vi "sCMOS_main.vi"   [LabVIEW 2015]
uses:
  CONTROLS/Q_camera_element.ctl
  CONTROLS/Q_main_element.ctl
  <vilib>/vision/Image Controls.llb/IMAQ Image.ctl
  CONTROLS/Global parameters.ctl
  GLOBAL/Global_CAMERA.vi
  GLOBAL/Global_ABORT.vi
  GLOBAL/Global_MAIN.vi
types:
  T1 = typedef "Q_main_element.ctl" = cluster{"variant":variant, "Instruction":enum16{"Main_idle", "Main_initialize", "Main_initialize_TDMS", "Main_initialize_Queue", "Main_error", "Main_DAQ_initialization_results", "Main_ASI_initialization_results", "Main_Piezo_initialization_results", "Main_Valve_initialization_results", "Main_Pump_initialization_results", "Main_CAMERA_initialization_results", "Main_DAQ_error", "Main_ASI_error", "Main_Piezo_error", "Main_CAMERA_error", "Main_Valve_error", "Main_Pump_error", "Main_start_acquiring", "Main_not_acquiring", "Main_acquiring", "Main_stop_acquiring", "Main_change_exposure", "Main_change_z_scan_parameters", "Main_define_ROI", "Main_read_kinetic_time", "Main_cooler", "Main_read_temperature", "Main_save_XY", "Main_define_mosaic", "Main_load_XY", "Main_discard_XY", "Main_move_to_XY", "Main_measure_QPD", "Main_autofocus_calibration", "Main_save_PID", "Main_change_H_valve_position", "Main_two_way_valve", "Main_save_movie", "Main_init_single_scan", "Main_single_scan", "Main_stop_single_scan", "Main_merFISH_illumination_parameters", "Main_merFISH_buffer_probe_list", "Main_merFISH_injections_procedure", "Main_merFISH_save_setpoint", "Main_merFISH_DAPI_parameters", "Main_merFISH_Brightfield_parameters", "Main_merFISH_save_embryo_ROI", "Main_merFISH_init", "Main_merFISH_resume", "Main_merFISH_start_autofocus", "Main_merFISH_open_close_valve_merFISH", "Main_merFISH_open_close_valve_photobleaching", "Main_merFISH_hybridization", "Main_merFISH_move_to_ROI", "Main_merFISH_wait_stabilization", "Main_merFISH_scan_laser", "Main_merFISH_scan_brightfield", "Main_merFISH_photobleaching_injection", "Main_merFISH_photobleaching", "Main_merFISH_save", "Main_merFISH_send_email", "Main_merFISH_close", "Main_TL_define_parameters", "Main_TL_FTL_reset_parameters", "Main_TL_init", "Main_TL_start_autofocus", "Main_TL_move_to_ROI", "Main_TL_wait_for_stabilization", "Main_TL_scan", "Main_TL_wait_cycle_end", "Main_TL_close", "Main_FTL_define_parameters", "Main_FTL_init", "Main_STOP"}}
  T2 = typedef "Image Type" = u32
  T3 = typedef "Q_camera_element.ctl" = cluster{"variant":variant, "Instruction":enum16{"CAMERA_idle", "CAMERA_initialize", "CAMERA_error", "CAMERA_security_stop", "CAMERA_not_acquiring", "CAMERA_acquiring", "CAMERA_start_acquiring", "CAMERA_stop_acquiring", "CAMERA_change_exposure", "CAMERA_define_ROI", "CAMERA_cooler", "CAMERA_acquire_movie", "CAMERA_init_scan", "CAMERA_check_new_scan_image", "CAMERA_close_scan", "CAMERA_init_merFISH", "CAMERA_start_acquiring_merFISH", "CAMERA_close_scan_merFISH", "CAMERA_close_merFISH", "CAMERA_init_TL", "CAMERA_start_acquiring_TL", "CAMERA_stop_acquiring_TL", "CAMERA_close_TL", "CAMERA_STOP"}}
  T4 = typedef "IMAQ Image.ctl" = refnum<image>
  T5 = cluster{"Total kinetic time (s)":dbl, "temperature":dbl, "coolerStatus":i32, "Error":bool, "Real time image":T4}
  T6 = cluster{"Exposure time":dbl, "Start acquisition":bool}
  T7 = cluster{"Sub Region":cluster{"Horizontal Offset":i32, "Vertical Offset":i32, "Horizontal Size":i32, "Vertical Size":i32}, "Start acquisition":bool}
  T8 = typedef "Global parameters.ctl" = cluster{"405":dbl, "488":dbl, "561":dbl, "641":dbl, "BF":dbl, "X":dbl, "Y":dbl, "Filter list":u16, "Exp time":sgl, "Kinetic time":sgl, "Gain":i32, "Step length (nm)":u32, "Total range (nm)":u32, "Scan illumination\n mode":bool, "Dt (s)":i32, "# repetitions":i32}
  T9 = cluster{"Saving path":path, "Sample name":string, "N frames":i32, "N movies":i32, "Start acquisition":bool, "Global parameters":T8}
  T10 = cluster{"Frames":i32, "Movie path":path, "Start acquisition":bool}
  T11 = cluster{"Pulse length Ton (s)":dbl, "image #":i32, "Display?":bool}
  T12 = cluster{"Mode":u32, "Polarity":u32, "Times":u32, "Delay":dbl}
  T13 = enum16{"CAMERA_idle", "CAMERA_initialize", "CAMERA_error", "CAMERA_security_stop", "CAMERA_not_acquiring", "CAMERA_acquiring", "CAMERA_start_acquiring", "CAMERA_stop_acquiring", "CAMERA_change_exposure", "CAMERA_define_ROI", "CAMERA_cooler", "CAMERA_acquire_movie", "CAMERA_init_scan", "CAMERA_check_new_scan_image", "CAMERA_close_scan", "CAMERA_init_merFISH", "CAMERA_start_acquiring_merFISH", "CAMERA_close_scan_merFISH", "CAMERA_close_merFISH", "CAMERA_init_TL", "CAMERA_start_acquiring_TL", "CAMERA_stop_acquiring_TL", "CAMERA_close_TL", "CAMERA_STOP"}
  T14 = cluster{"Horizontal Offset":i32, "Vertical Offset":i32, "Horizontal Size":i32, "Vertical Size":i32}
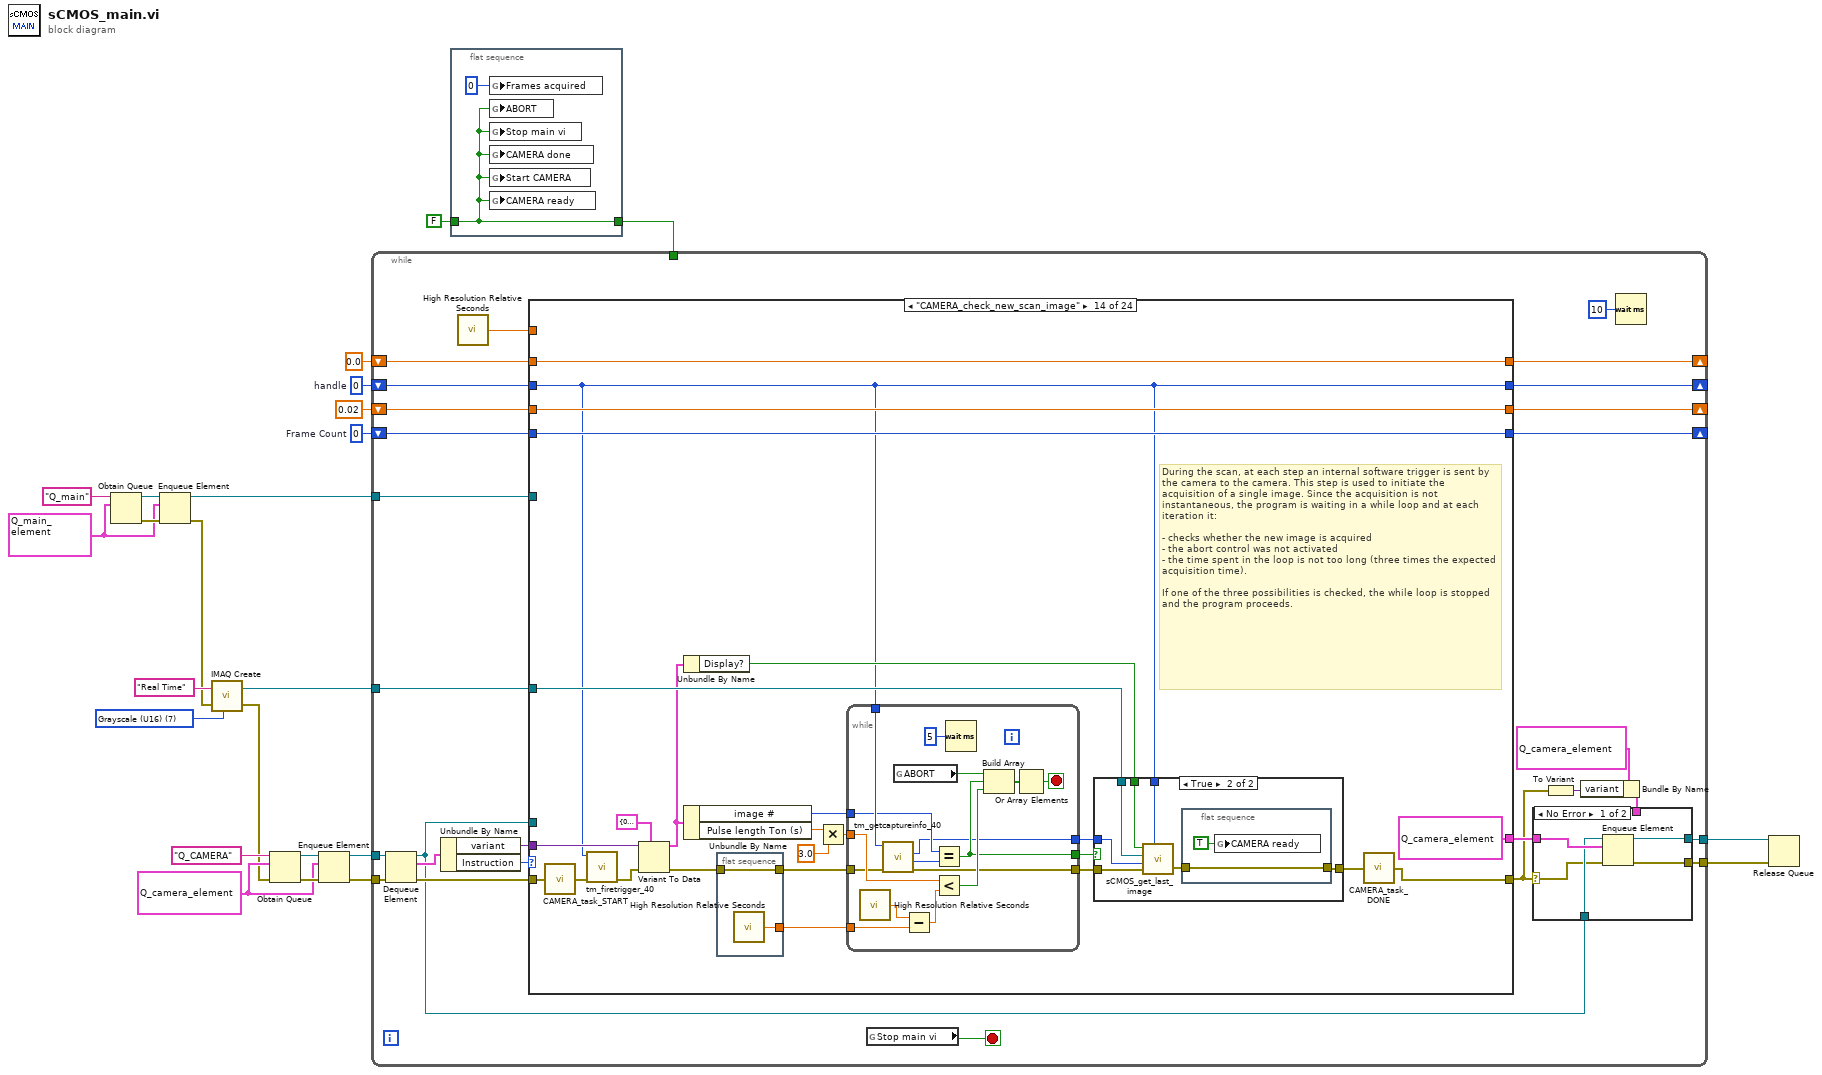
[diagram p0: block diagram]
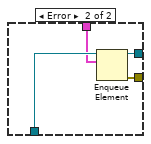
[diagram p2: hidden frame]
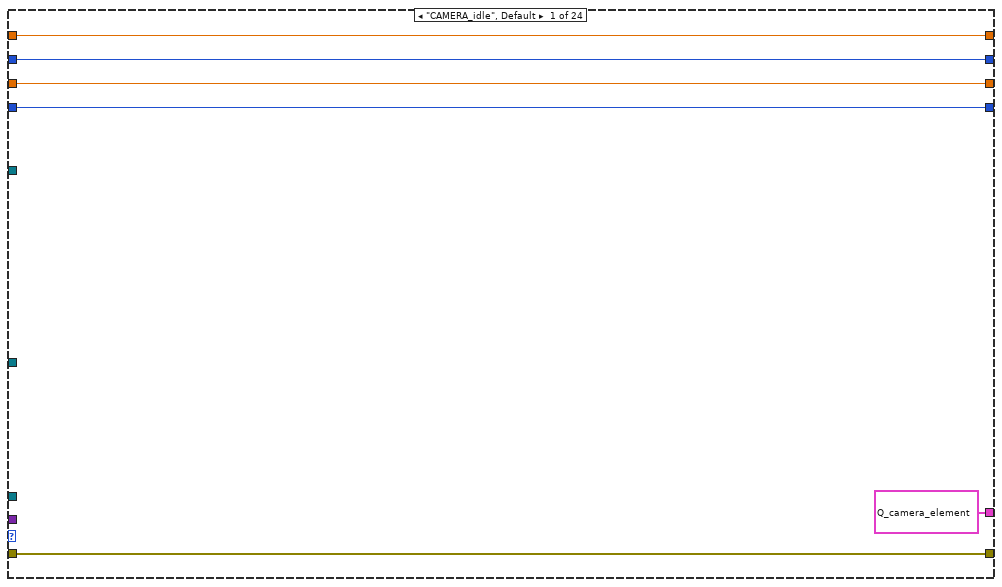
[diagram p3: hidden frame]
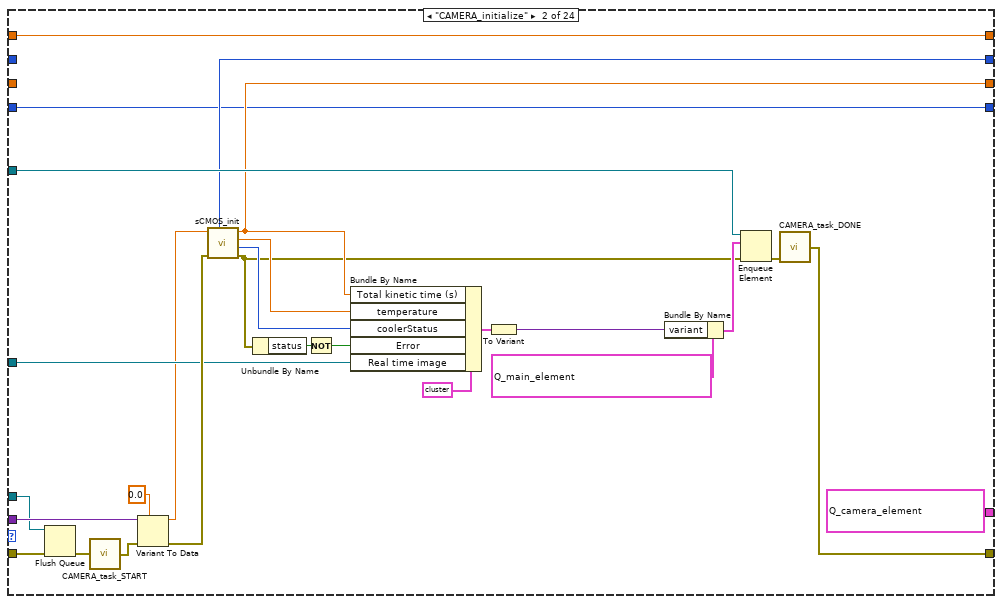
[diagram p4: hidden frame]
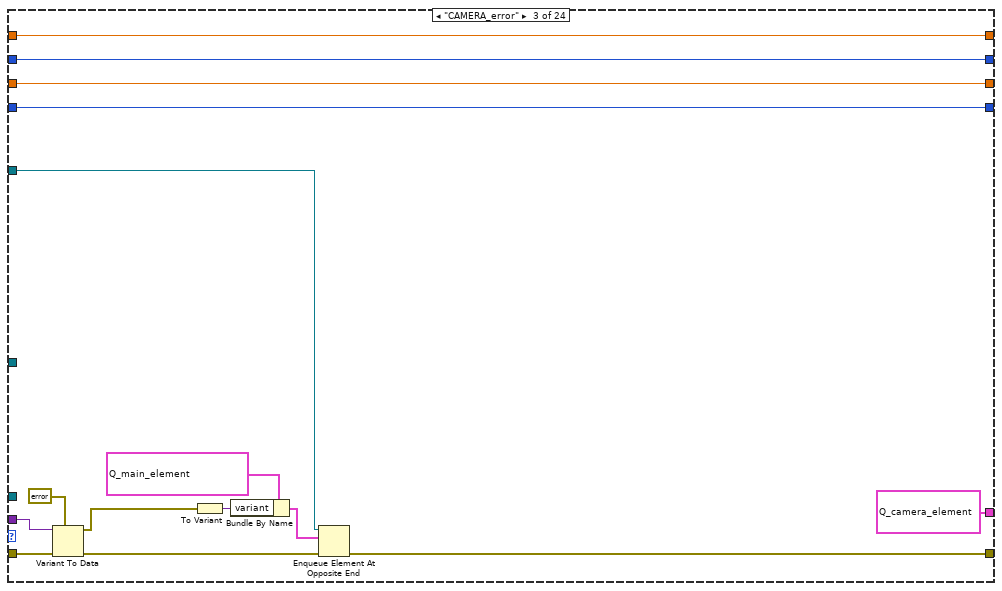
[diagram p5: hidden frame]
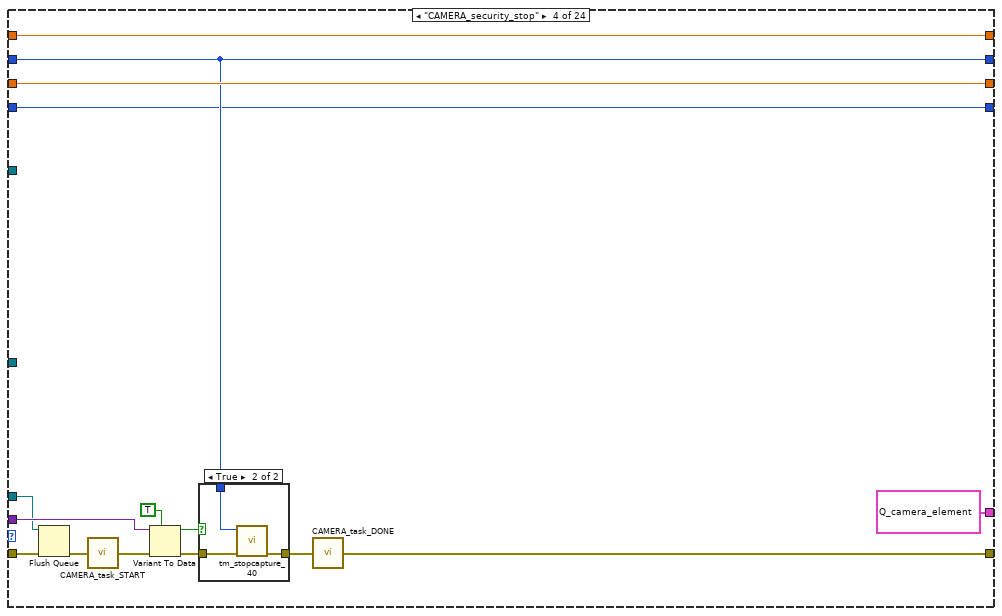
[diagram p6: hidden frame]
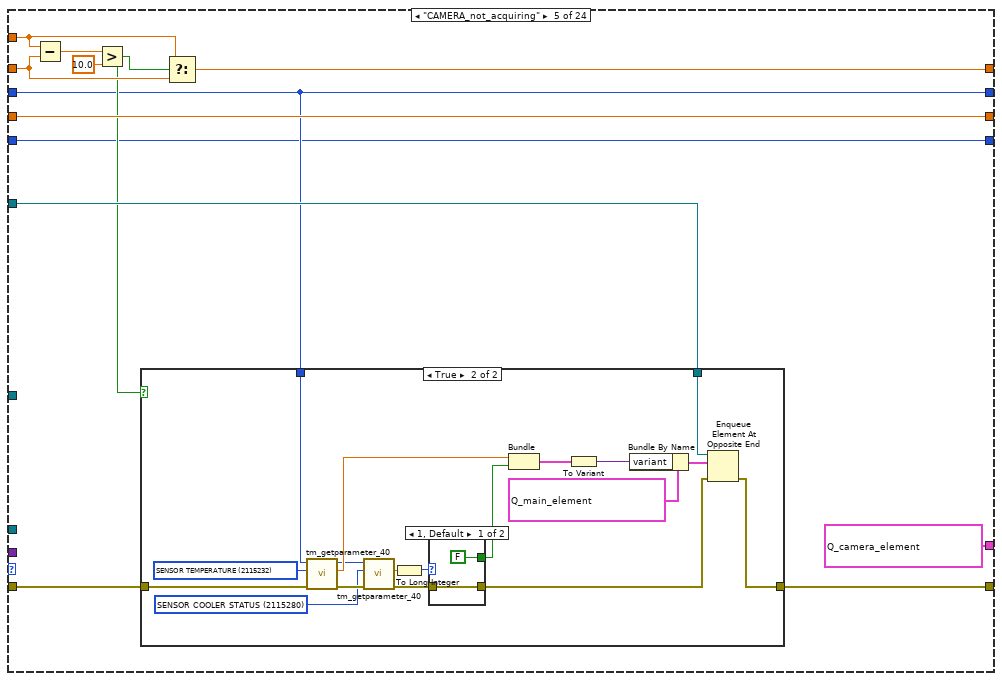
[diagram p8: hidden frame]
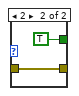
[diagram p10: hidden frame]
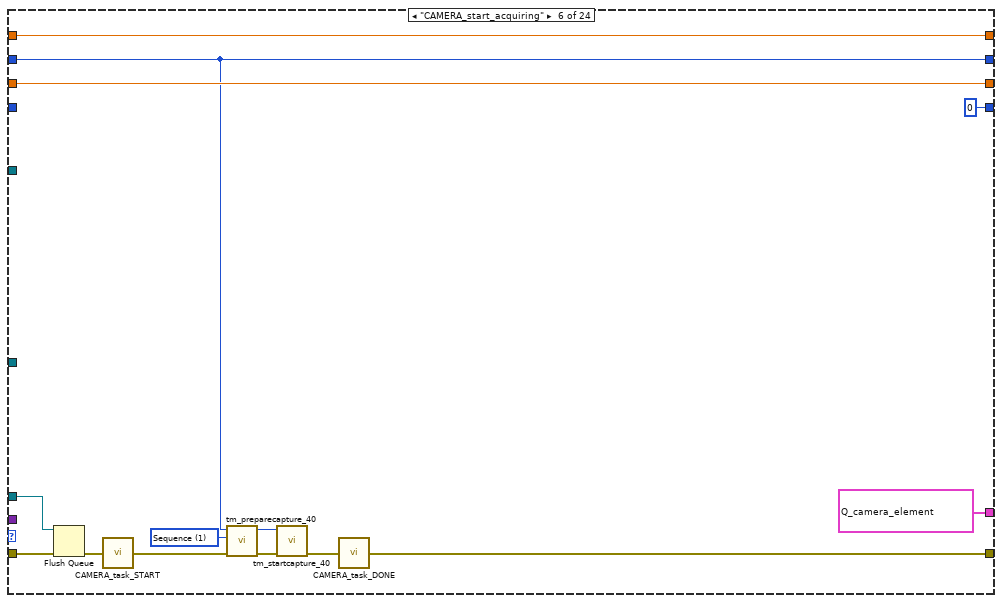
[diagram p11: hidden frame]
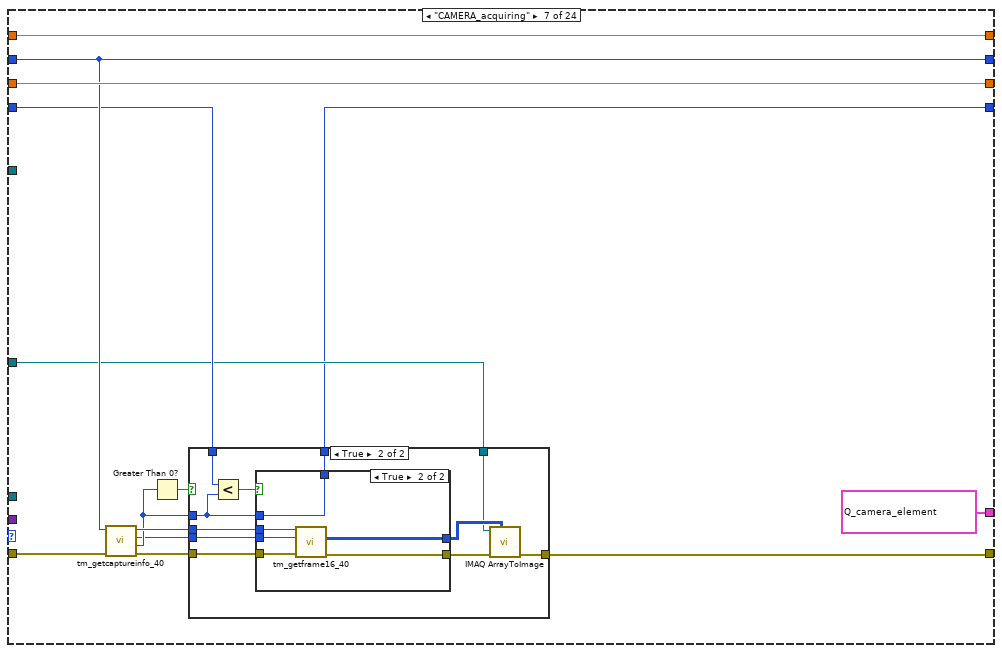
[diagram p12: hidden frame]
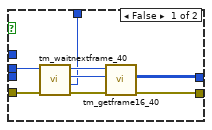
[diagram p14: hidden frame]
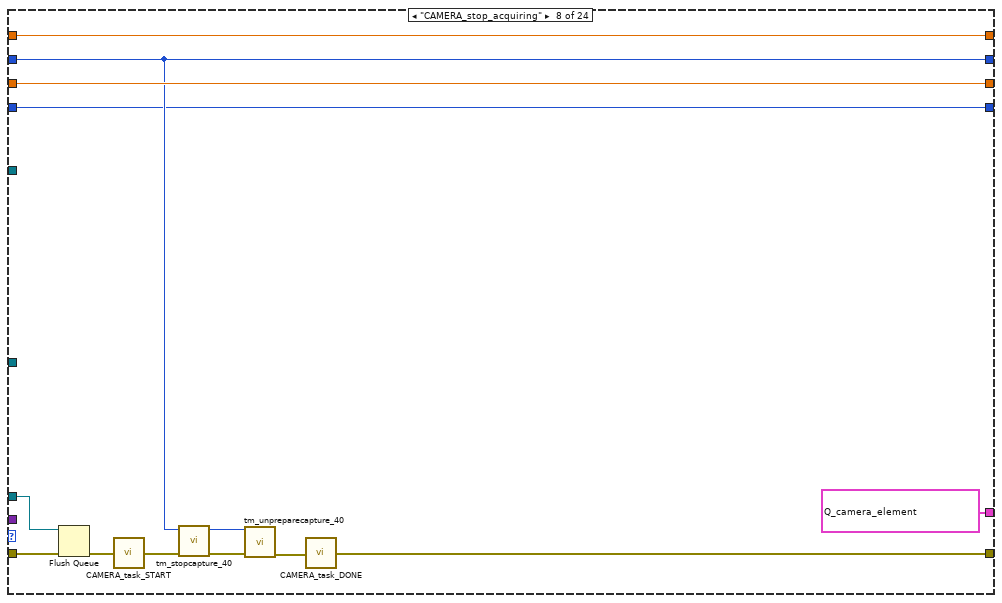
[diagram p15: hidden frame]
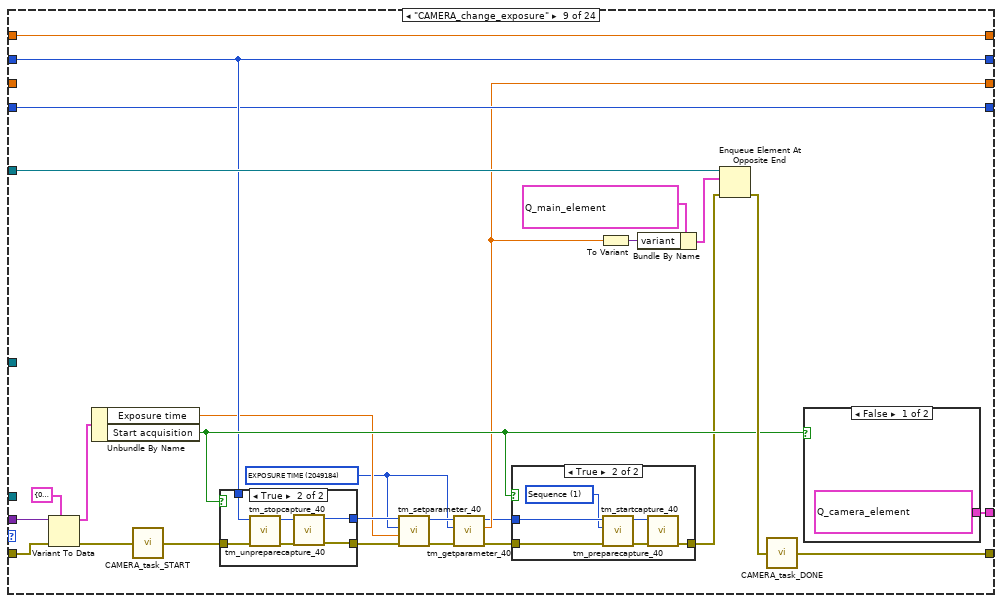
[diagram p16: hidden frame]
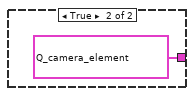
[diagram p18: hidden frame]
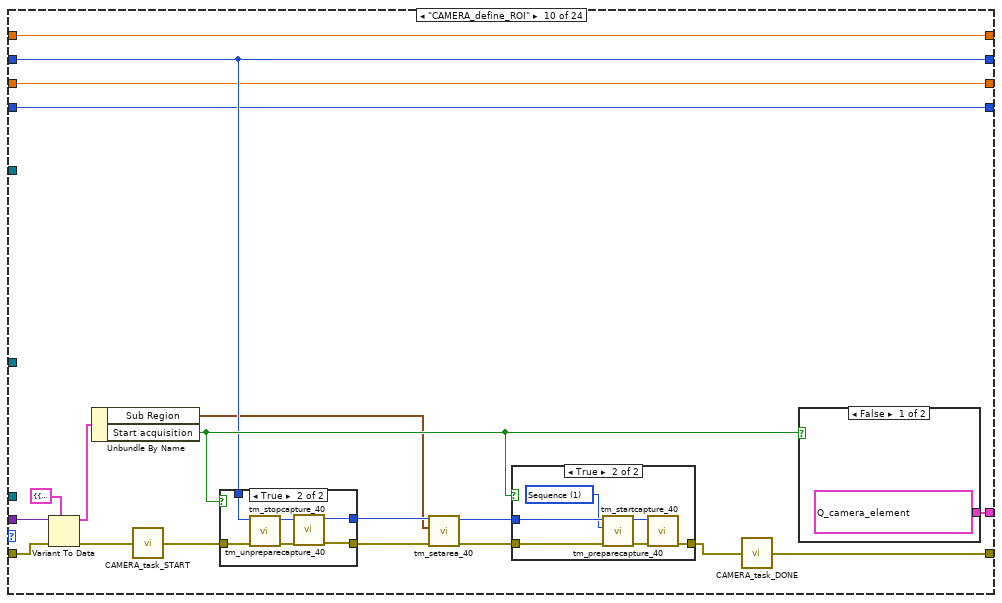
[diagram p20: hidden frame]
diagram:
  w1 = 0  # Frame Count
  w2 = u32 0  # handle
  w3 = T1 {"variant"=variant, "Instruction"=enum."Main_idle"} ("Q_main_element")
  w14 = T2 7 items=["Grayscale (U8)", "Grayscale (I16)", "Grayscale (SGL)", "Complex (CSG)", "RGB (U32)", "HSL (U32)", "RGB (U64)", "Grayscale (U16)"] ("Image Type")
  w19 = T3 {"variant"=variant, "Instruction"=enum."CAMERA_idle"} ("Q_ANDOR_element")
  n1 = Obtain Queue(name (unnamed)="Q_main", element data type=w3) -> (queue out=w17:refnum<queue>, error out=w18:errorcluster)  [unwired: 3 in, 1 out]
  n2 = Enqueue Element(queue=w17, element=w3, error in (no error)=w18) -> (queue out=w16:refnum<queue>, error out=w13:errorcluster)  [unwired: 1 in, 1 out]
  n3 = call "IMAQ Create"("Image Name"="Real Time", "Image Type"=w14, "error in (no error)"=w13) -> ("New Image"=w12:T4, "error out"=w9:errorcluster)  [unwired: 2 in]
  n4 = Obtain Queue(name (unnamed)="Q_CAMERA", element data type=w19, error in (no error)=w9) -> (queue out=w23:refnum<queue>, error out=w22:errorcluster)  [unwired: 2 in, 1 out]
  n5 = Enqueue Element(queue=w23, element=w19, error in (no error)=w22) -> (queue out=w21:refnum<queue>, error out=w20:errorcluster)  [unwired: 1 in, 1 out]
  n6 = while {
    tunnel: w21 -> [w50]
    tunnel: w20 -> [w49]
    tunnel: [w44] -> w6
    tunnel: w16 -> [w43]
    tunnel: w12 -> [w41]
    shift-right: [w39] -> _
    shift-left: 0.02 -> [w40]
    shift-right: [w38] -> _
    shift-left: 0.0 ("Period") -> [w37]
    tunnel: w7 -> [_]
    tunnel: [w36] -> w5
    shift-right: [w30] -> _
    shift-left: w2 -> [w31]
    shift-right: [w28] -> _
    shift-left: w1 -> [w29]
    stop <- w51 stop-if-true
    n7 = Dequeue Element(queue=w50, error in (no error)=w49) -> (queue out=w25:refnum<queue>, element=w48:T3, error out=w46:errorcluster)  [unwired: 1 in, 1 out]
    n8 = Unbundle By Name(w48) -> ("variant"=w42:variant, "Instruction"=w47:T13)
    n9 = call <vilib>:"High Resolution Relative Seconds.vi"() -> ("relative seconds"=w27:dbl)
    n10 = case shown="\"CAMERA_check_new_scan_image\"" w47 {
      tunnel: w46 -> [w64 w79 w107 w111 w138 w173 w188 w228 w257 w293 w328 w347 w398 w424 w474 w490 w510 w529 w548 w566 w591 w610 w632 w650]
      tunnel: [w64 w75 w94 w120 w137 w174 w180 w227 w250 w289 w323 w345 w397 w416 w475 w489 w513 w530 w549 w565 w590 w609 w633 w648] -> w33
      tunnel: [T3 {"variant"=variant, "Instruction"=enum."CAMERA_idle"} ("Q_ANDOR_element") T3 {"variant"=variant, "Instruction"=enum."CAMERA_not_acquiring"} ("Q_ANDOR_element") T3 {"variant"=variant, "Instruction"=enum."CAMERA_idle"} ("Q_ANDOR_element") T3 {"variant"=variant, "Instruction"=enum."CAMERA_idle"} ("Q_ANDOR_element") T3 {"variant"=variant, "Instruction"=enum."CAMERA_not_acquiring"} ("Q_ANDOR_element") T3 {"variant"=variant, "Instruction"=enum."CAMERA_acquiring"} ("Q_ANDOR_element") T3 {"variant"=variant, "Instruction"=enum."CAMERA_acquiring"} ("Q_ANDOR_element") T3 {"variant"=variant, "Instruction"=enum."CAMERA_not_acquiring"} ("Q_ANDOR_element") w248 w287 T3 {"variant"=variant, "Instruction"=enum."CAMERA_not_acquiring"} ("Q_ANDOR_element") T3 {"variant"=variant, "Instruction"=enum."CAMERA_idle"} ("Q_ANDOR_element") T3 {"variant"=variant, "Instruction"=enum."CAMERA_idle"} ("Q_ANDOR_element") T3 {"variant"=variant, "Instruction"=enum."CAMERA_idle"} ("Q_ANDOR_element") T3 {"variant"=variant, "Instruction"=enum."CAMERA_idle"} ("Q_ANDOR_element") T3 {"variant"=variant, "Instruction"=enum."CAMERA_idle"} ("Q_ANDOR_element") T3 {"variant"=variant, "Instruction"=enum."CAMERA_idle"} ("Q_ANDOR_element") T3 {"variant"=variant, "Instruction"=enum."CAMERA_idle"} ("Q_ANDOR_element") T3 {"variant"=variant, "Instruction"=enum."CAMERA_idle"} ("Q_ANDOR_element") T3 {"variant"=variant, "Instruction"=enum."CAMERA_idle"} ("Q_ANDOR_element") T3 {"variant"=variant, "Instruction"=enum."CAMERA_idle"} ("Q_ANDOR_element") T3 {"variant"=variant, "Instruction"=enum."CAMERA_idle"} ("Q_ANDOR_element") T3 {"variant"=variant, "Instruction"=enum."CAMERA_idle"} ("Q_ANDOR_element") T3 {"variant"=variant, "Instruction"=enum."CAMERA_idle"} ("Q_ANDOR_element")] -> w45
      tunnel: w43 -> [_ w92 w101 _ w134 _ _ _ w253 _ _ _ _ _ _ _ _ _ _ _ _ _ _ _]
      tunnel: w42 -> [_ w89 w108 w116 _ _ _ _ w258 w294 w327 w352 w399 w423 _ w491 w507 _ _ w567 w582 _ _ w640]
      tunnel: w41 -> [_ w83 _ _ _ _ w179 _ _ _ _ w349 _ w421 _ _ _ _ _ _ _ _ _ w647]
      tunnel: [w65 w76 w97 w121 w139 w177 w191 w230 w234 w283 w325 w350 w395 w418 w472 0.05000000074505806 ("kinetic") w516 w527 w531 0.05000000074505806 ("kinetic") 0.05000000074505806 ("kinetic") 0.05000000074505806 ("kinetic") w615 w651] -> w39
      tunnel: w40 -> [w65 _ w97 w121 w139 w177 w191 w230 _ w283 w325 w350 w395 w418 w472 _ w516 w527 w531 _ _ _ w615 w651]
      tunnel: w37 -> [w66 w86 w98 w122 w133 w176 w190 w229 w247 w286 w315 w351 w396 w417 w473 w487 w515 w528 w547 w563 w588 w607 w631 w649]
      tunnel: [w66 w86 w98 w122 w131 w176 w190 w229 w247 w286 w315 w351 w396 w417 w473 w487 w515 w528 w547 w563 w588 w607 w631 w649] -> w38
      tunnel: w27 -> [_ _ _ _ w132 _ _ _ _ _ _ _ _ _ _ _ _ _ _ _ _ _ _ _]
      tunnel: w25 -> [_ w77 _ w109 _ w171 _ w225 _ _ _ _ w391 _ _ w483 w512 _ _ w559 _ _ _ w636]
      tunnel: w31 -> [w62 _ w96 w118 w129 w169 w187 w223 w246 w285 w314 w339 w386 w400 w456 w479 w496 w520 w532 w555 w576 w603 w616 w645]
      tunnel: [w62 w70 w96 w118 w129 w169 w187 w223 w246 w285 w314 w339 w386 w400 w456 w479 w496 w520 w532 w555 w576 w603 w616 w645] -> w30
      tunnel: w29 -> [w61 w69 w95 w117 w128 _ w182 w222 w245 w284 w312 w342 w388 w415 w470 w481 w511 w525 w544 w557 w585 w604 w628 w646]
      tunnel: [w61 w69 w95 w117 w128 0 ("Frame Count") w178 w222 w245 w284 w312 w342 w388 w415 w470 w481 w511 w525 w544 w557 w585 w604 w628 w646] -> w28
      frame "CAMERA_idle", Default {
      }
      frame "CAMERA_initialize" {
        n11 = Flush Queue(queue=w77, error in (no error)=w79) -> (error out=w78:errorcluster)  [unwired: 2 out]
        n12 = call "CAMERA_task_START.vi"("error in"=w78) -> ("error out"=w82:errorcluster)
        n13 = Variant To Data(error in=w82, type=0.0, Variant=w89) -> (data=w73:dbl, error out=w88:errorcluster)
        n14 = call "sCMOS_init.vi"("error in"=w88, "Exposure time"=w73) -> ("error out"=w67:errorcluster, "Cooler status"=w72:i32, "temperature"=w71:dbl, "Exposure time out"=w76:dbl, "Handle out"=w70:u32)  [unwired: 2 in]
        n15 = Unbundle By Name(w67) -> ("status"=w90:bool)
        n16 = Not(x=w90) -> (.not. x?=w87:bool)
        n17 = Bundle By Name(cluster=T5 {"Total kinetic time (s)"=0.0, "temperature"=0.0, "coolerStatus"=0, "Error"=FALSE, "Real time image"=refnum}, "Total kinetic time (s)"=w76, "temperature"=w71, "coolerStatus"=w72, "Error"=w87, "Real time image"=w83) -> (w84:T5)
        n18 = To Variant(anything=w84) -> (Variant=w91:variant)
        n19 = Bundle By Name(cluster=T1 {"variant"=variant, "Instruction"=enum."Main_CAMERA_initialization_results"} ("Q_main_element"), "variant"=w91) -> (w80:T1)
        n20 = Enqueue Element(queue=w92, element=w80, error in (no error)=w67) -> (error out=w68:errorcluster)  [unwired: 1 in, 2 out]
        n21 = call "CAMERA_task_DONE.vi"("error in"=w68) -> ("error out"=w75:errorcluster)
      }
      frame "CAMERA_error" {
        n22 = Variant To Data(error in=w107, type=errorcluster {"status"=FALSE, "code"=0, "source"=""} ("error out"), Variant=w108) -> (data=w103:errorcluster, error out=w100:errorcluster)
        n23 = To Variant(anything=w103) -> (Variant=w104:variant)
        n24 = Bundle By Name(cluster=T1 {"variant"=variant, "Instruction"=enum."Main_CAMERA_error"} ("Q_main_element"), "variant"=w104) -> (w102:T1)
        n25 = Enqueue Element At Opposite End(queue=w101, element=w102, error in (no error)=w100) -> (error out=w94:errorcluster)  [unwired: 1 in, 2 out]
      }
      frame "CAMERA_security_stop" {
        n26 = Flush Queue(queue=w109, error in (no error)=w111) -> (error out=w110:errorcluster)  [unwired: 2 out]
        n27 = call "CAMERA_task_START.vi"("error in"=w110) -> ("error out"=w112:errorcluster)
        n28 = Variant To Data(error in=w112, type=TRUE, Variant=w116) -> (data=w114:bool, error out=w113:errorcluster)
        n29 = case shown="True" w114 {
          tunnel: [w124 w127] -> w119
          tunnel: w118 -> [_ w126]
          tunnel: w113 -> [w124 w125]
          frame False {
          }
          frame True {
            n30 = call <userlib>:"tm_stopcapture_40.vi"("error in (no error)"=w125, "Handle in"=w126) -> ("error out"=w127:errorcluster)  [unwired: 8 in, 1 out]
          }
        }
        n31 = call "CAMERA_task_DONE.vi"("error in"=w119) -> ("error out"=w120:errorcluster)
      }
      frame "CAMERA_not_acquiring" {
        n32 = Subtract(x=w132, y=w133) -> (x-y=w136:dbl)
        n33 = Greater?(x=w136, y=10.0) -> (0:w130:bool)
        n34 = case shown="True" w130 {
          tunnel: w138 -> [w141 w152]
          tunnel: [w141 w159] -> w137
          tunnel: w134 -> [_ w158]
          tunnel: w129 -> [_ w151]
          frame False {
          }
          frame True {
            w146 = u32 2115280 items=["SENSOR MODE"=4212128, "READOUT SPEED"=4211872, "READOUT DIRECTION"=4211904, "TRIGGER GLOBAL EXPOSURE"=2049680, "TRIGGER DELAY"=1066480, "INTERNAL TRIGGER HANDLING"=1066496, "SYNC READOUT SYSTEM BLANK"=1066528, "SENSOR TEMPERATURE"=2115232, "SENSOR COOLER STATUS"=2115280, "EXPOSURE TIME"=2049184, "DEFECT CORRECT MODE"=4670368, "BINNING"=4215968, "INTERNAL LINE SPEED"=4226000, "INTERNAL LINE INTERVAL"=4226016, "NUMBER OF OUTPUT TRIGGER CONNECTOR"=1852320, "OUTPUT TRIGGER SOURCE[0]"=1852576, "OUTPUT TRIGGER SOURCE[1]"=1852832, "OUTPUT TRIGGER SOURCE[2]"=1853088, "OUTPUT TRIGGER POLARITY[0]"=1852592, "OUTPUT TRIGGER POLARITY[1]"=1852848, "OUTPUT TRIGGER POLARITY[2]"=1853104, "OUTPUT TRIGGER ACTIVE[0]"=1852608, "OUTPUT TRIGGER ACTIVE[1]"=1852864, "OUTPUT TRIGGER ACTIVE[2]"=1853120, "OUTPUT TRIGGER DELAY[0]"=1852624, "OUTPUT TRIGGER DELAY[1]"=1852880, "OUTPUT TRIGGER DELAY[2]"=1853136, "OUTPUT TRIGGER PERIOD[0]"=1852640, "OUTPUT TRIGGER PERIOD[1]"=1852896, "OUTPUT TRIGGER PERIOD[2]"=1853152, "OUTPUT TRIGGER KIND[0]"=1852656, "OUTPUT TRIGGER KIND[1]"=1852912, "OUTPUT TRIGGER KIND[2]"=1853168, "OUTPUT TRIGGER BASE SENSOR[0]"=1852672, "OUTPUT TRIGGER BASE SENSOR[1]"=1852928, "OUTPUT TRIGGER BASE SENSOR[2]"=1853184, "OUTPUT TRIGGER PRE HSYNC COUNT"=1852704] ("Parameter")
            w150 = u32 2115232 items=["SENSOR MODE"=4212128, "READOUT SPEED"=4211872, "READOUT DIRECTION"=4211904, "TRIGGER GLOBAL EXPOSURE"=2049680, "TRIGGER DELAY"=1066480, "INTERNAL TRIGGER HANDLING"=1066496, "SYNC READOUT SYSTEM BLANK"=1066528, "SENSOR TEMPERATURE"=2115232, "SENSOR COOLER STATUS"=2115280, "EXPOSURE TIME"=2049184, "DEFECT CORRECT MODE"=4670368, "BINNING"=4215968, "INTERNAL LINE SPEED"=4226000, "INTERNAL LINE INTERVAL"=4226016, "NUMBER OF OUTPUT TRIGGER CONNECTOR"=1852320, "OUTPUT TRIGGER SOURCE[0]"=1852576, "OUTPUT TRIGGER SOURCE[1]"=1852832, "OUTPUT TRIGGER SOURCE[2]"=1853088, "OUTPUT TRIGGER POLARITY[0]"=1852592, "OUTPUT TRIGGER POLARITY[1]"=1852848, "OUTPUT TRIGGER POLARITY[2]"=1853104, "OUTPUT TRIGGER ACTIVE[0]"=1852608, "OUTPUT TRIGGER ACTIVE[1]"=1852864, "OUTPUT TRIGGER ACTIVE[2]"=1853120, "OUTPUT TRIGGER DELAY[0]"=1852624, "OUTPUT TRIGGER DELAY[1]"=1852880, "OUTPUT TRIGGER DELAY[2]"=1853136, "OUTPUT TRIGGER PERIOD[0]"=1852640, "OUTPUT TRIGGER PERIOD[1]"=1852896, "OUTPUT TRIGGER PERIOD[2]"=1853152, "OUTPUT TRIGGER KIND[0]"=1852656, "OUTPUT TRIGGER KIND[1]"=1852912, "OUTPUT TRIGGER KIND[2]"=1853168, "OUTPUT TRIGGER BASE SENSOR[0]"=1852672, "OUTPUT TRIGGER BASE SENSOR[1]"=1852928, "OUTPUT TRIGGER BASE SENSOR[2]"=1853184, "OUTPUT TRIGGER PRE HSYNC COUNT"=1852704] ("Parameter")
            n35 = call <userlib>:"tm_getparameter_40.vi"("error in (no error)"=w152, "Parameter"=w150, "Handle in"=w151) -> ("error out"=w148:errorcluster, "Value out"=w149:dbl, "Handle out"=w147:u32)  [unwired: 6 in]
            n36 = call <userlib>:"tm_getparameter_40.vi"("error in (no error)"=w148, "Parameter"=w146, "Handle in"=w147) -> ("error out"=w144:errorcluster, "Value out"=w145:dbl)  [unwired: 6 in, 1 out]
            n37 = To Long Integer(number=w145) -> (32bit integer=w142:i32)
            n38 = case shown="1, Default" w142 {
              tunnel: [FALSE TRUE] -> w155
              tunnel: w144 -> [w160 w162]
              tunnel: [w160 w162] -> w143
              frame 1, Default {
              }
              frame 2 {
              }
            }
            n39 = Bundle("Value out"=w149, w155) -> (w154:cluster{"Value out":dbl, bool})  [unwired: 1 in]
            n40 = To Variant(anything=w154) -> (Variant=w156:variant)
            n41 = Bundle By Name(cluster=T1 {"variant"=variant, "Instruction"=enum."Main_read_temperature"} ("Q_main_element"), "variant"=w156) -> (w153:T1)
            n42 = Enqueue Element At Opposite End(queue=w158, element=w153, error in (no error)=w143) -> (error out=w159:errorcluster)  [unwired: 1 in, 2 out]
          }
        }
        n43 = Select(t=w132, s=w130, f=w133) -> (s? t:f=w131:dbl)
      }
      frame "CAMERA_start_acquiring" {
        w168 = 1 items=["Snap", "Sequence"] ("Capture mode")
        n44 = Flush Queue(queue=w171, error in (no error)=w173) -> (error out=w172:errorcluster)  [unwired: 2 out]
        n45 = call "CAMERA_task_START.vi"("error in"=w172) -> ("error out"=w170:errorcluster)
        n46 = call <userlib>:"tm_preparecapture_40.vi"("error in (no error)"=w170, "Capture mode"=w168, "Handle in"=w169) -> ("error out"=w167:errorcluster, "Handle out"=w166:u32)  [unwired: 5 in, 2 out]
        n47 = call <userlib>:"tm_startcapture_40.vi"("error in (no error)"=w167, "Handle in"=w166) -> ("error out"=w165:errorcluster)  [unwired: 8 in, 1 out]
        n48 = call "CAMERA_task_DONE.vi"("error in"=w165) -> ("error out"=w174:errorcluster)
      }
      frame "CAMERA_acquiring" {
        n49 = call <userlib>:"tm_getcaptureinfo_40.vi"("error in (no error)"=w188, "Handle in"=w187) -> ("error out"=w184:errorcluster, "Frame Count"=w183:i32, "Frame Index"=w181:i32, "Handle out"=w185:u32)  [unwired: 6 in]
        n50 = Greater Than 0?(x=w183) -> (x > 0?=w186:bool)
        n51 = case shown="True" w186 {
          tunnel: w185 -> [_ w202]
          tunnel: w184 -> [w193 w201]
          tunnel: w183 -> [w192 w194]
          tunnel: w182 -> [_ w204]
          tunnel: w181 -> [_ w200]
          tunnel: [w193 w197] -> w180
          tunnel: w179 -> [_ w196]
          tunnel: [w192 w195] -> w178
          frame False {
          }
          frame True {
            n52 = Less?(x=w204, y=w194) -> (x < y?=w203:bool)
            n53 = case shown="True" w203 {
              tunnel: w202 -> [w211 w218]
              tunnel: w201 -> [w212 w217]
              tunnel: w200 -> [_ w216]
              tunnel: [w206 w215] -> w199
              tunnel: [w207 w214] -> w198
              tunnel: [w205 w213] -> w195
              tunnel: w194 -> [_ w213]
              frame False {
                n54 = call <userlib>:"tm_waitnextframe_40.vi"("error in (no error)"=w212, "Handle in"=w211) -> ("error out"=w210:errorcluster, "Frame Count"=w205:i32, "Frame Index"=w209:i32, "Handle out"=w208:u32)  [unwired: 6 in]
                n55 = call <userlib>:"tm_getframe16_40.vi"("error in (no error)"=w210, "Frame Index"=w209, "Handle in"=w208) -> ("error out"=w206:errorcluster, "Data"=w207:u16[][])  [unwired: 5 in, 2 out]
              }
              frame True {
                n56 = call <userlib>:"tm_getframe16_40.vi"("error in (no error)"=w217, "Frame Index"=w216, "Handle in"=w218) -> ("error out"=w215:errorcluster, "Data"=w214:u16[][])  [unwired: 5 in, 2 out]
              }
            }
            n57 = call "IMAQ ArrayToImage"("Image Pixels (U16)"=w198, "error in (no error)"=w199, "Image"=w196) -> ("error out"=w197:errorcluster)  [unwired: 7 in, 1 out]
          }
        }
      }
      frame "CAMERA_stop_acquiring" {
        n58 = Flush Queue(queue=w225, error in (no error)=w228) -> (error out=w226:errorcluster)  [unwired: 2 out]
        n59 = call "CAMERA_task_START.vi"("error in"=w226) -> ("error out"=w224:errorcluster)
        n60 = call <userlib>:"tm_stopcapture_40.vi"("error in (no error)"=w224, "Handle in"=w223) -> ("error out"=w220:errorcluster, "Handle out"=w221:u32)  [unwired: 8 in]
        n61 = call <userlib>:"tm_unpreparecapture_40.vi"("error in (no error)"=w220, "Handle in"=w221) -> ("error out"=w219:errorcluster)  [unwired: 8 in, 1 out]
        n62 = call "CAMERA_task_DONE.vi"("error in"=w219) -> ("error out"=w227:errorcluster)
      }
      frame "CAMERA_change_exposure" {
        w235 = u32 2049184 items=["SENSOR MODE"=4212128, "READOUT SPEED"=4211872, "READOUT DIRECTION"=4211904, "TRIGGER GLOBAL EXPOSURE"=2049680, "TRIGGER DELAY"=1066480, "INTERNAL TRIGGER HANDLING"=1066496, "SYNC READOUT SYSTEM BLANK"=1066528, "SENSOR TEMPERATURE"=2115232, "SENSOR COOLER STATUS"=2115280, "EXPOSURE TIME"=2049184, "DEFECT CORRECT MODE"=4670368, "BINNING"=4215968, "INTERNAL LINE SPEED"=4226000, "INTERNAL LINE INTERVAL"=4226016, "NUMBER OF OUTPUT TRIGGER CONNECTOR"=1852320, "OUTPUT TRIGGER SOURCE[0]"=1852576, "OUTPUT TRIGGER SOURCE[1]"=1852832, "OUTPUT TRIGGER SOURCE[2]"=1853088, "OUTPUT TRIGGER POLARITY[0]"=1852592, "OUTPUT TRIGGER POLARITY[1]"=1852848, "OUTPUT TRIGGER POLARITY[2]"=1853104, "OUTPUT TRIGGER ACTIVE[0]"=1852608, "OUTPUT TRIGGER ACTIVE[1]"=1852864, "OUTPUT TRIGGER ACTIVE[2]"=1853120, "OUTPUT TRIGGER DELAY[0]"=1852624, "OUTPUT TRIGGER DELAY[1]"=1852880, "OUTPUT TRIGGER DELAY[2]"=1853136, "OUTPUT TRIGGER PERIOD[0]"=1852640, "OUTPUT TRIGGER PERIOD[1]"=1852896, "OUTPUT TRIGGER PERIOD[2]"=1853152, "OUTPUT TRIGGER KIND[0]"=1852656, "OUTPUT TRIGGER KIND[1]"=1852912, "OUTPUT TRIGGER KIND[2]"=1853168, "OUTPUT TRIGGER BASE SENSOR[0]"=1852672, "OUTPUT TRIGGER BASE SENSOR[1]"=1852928, "OUTPUT TRIGGER BASE SENSOR[2]"=1853184, "OUTPUT TRIGGER PRE HSYNC COUNT"=1852704] ("Parameter")
        n63 = Variant To Data(error in=w257, type=T6 {"Exposure time"=0.0, "Start acquisition"=FALSE} ("output cluster"), Variant=w258) -> (data=w254:T6, error out=w256:errorcluster)
        n64 = Unbundle By Name(w254) -> ("Exposure time"=w238:dbl, "Start acquisition"=w249:bool)
        n65 = call "CAMERA_task_START.vi"("error in"=w256) -> ("error out"=w251:errorcluster)
        n66 = case shown="True" w249 {
          tunnel: [w269 w271] -> w240
          tunnel: w251 -> [w269 w275]
          tunnel: w246 -> [w268 w274]
          tunnel: [w268 w270] -> w239
          frame False {
          }
          frame True {
            n67 = call <userlib>:"tm_stopcapture_40.vi"("error in (no error)"=w275, "Handle in"=w274) -> ("error out"=w273:errorcluster, "Handle out"=w272:u32)  [unwired: 8 in]
            n68 = call <userlib>:"tm_unpreparecapture_40.vi"("error in (no error)"=w273, "Handle in"=w272) -> ("error out"=w271:errorcluster, "Handle out"=w270:u32)  [unwired: 8 in]
          }
        }
        n69 = call <userlib>:"tm_setparameter_40.vi"("error in (no error)"=w240, "Value in"=w238, "Parameter"=w235, "Handle in"=w239) -> ("error out"=w237:errorcluster, "Handle out"=w236:u32)  [unwired: 6 in]
        n70 = call <userlib>:"tm_getparameter_40.vi"("error in (no error)"=w237, "Parameter"=w235, "Handle in"=w236) -> ("error out"=w233:errorcluster, "Value out"=w234:dbl, "Handle out"=w232:u32)  [unwired: 6 in]
        n71 = case shown="True" w249 {
          tunnel: w233 -> [w259 w265]
          tunnel: [w259 w260] -> w241
          tunnel: w232 -> [_ w264]
          frame False {
          }
          frame True {
            w263 = 1 items=["Snap", "Sequence"] ("Capture mode")
            n72 = call <userlib>:"tm_preparecapture_40.vi"("error in (no error)"=w265, "Capture mode"=w263, "Handle in"=w264) -> ("error out"=w262:errorcluster, "Handle out"=w261:u32)  [unwired: 5 in, 2 out]
            n73 = call <userlib>:"tm_startcapture_40.vi"("error in (no error)"=w262, "Handle in"=w261) -> ("error out"=w260:errorcluster)  [unwired: 8 in, 1 out]
          }
        }
        n74 = To Variant(anything=w234) -> (Variant=w243:variant)
        n75 = Bundle By Name(cluster=T1 {"variant"=variant, "Instruction"=enum."Main_read_kinetic_time"} ("Q_main_element"), "variant"=w243) -> (w244:T1)
        n76 = Enqueue Element At Opposite End(queue=w253, element=w244, error in (no error)=w241) -> (error out=w252:errorcluster)  [unwired: 1 in, 2 out]
        n77 = call "CAMERA_task_DONE.vi"("error in"=w252) -> ("error out"=w250:errorcluster)
        n78 = case shown="False" w249 {
          tunnel: [T3 {"variant"=variant, "Instruction"=enum."CAMERA_not_acquiring"} ("Q_ANDOR_element") T3 {"variant"=variant, "Instruction"=enum."CAMERA_acquiring"} ("Q_ANDOR_element")] -> w248
          frame False {
          }
          frame True {
          }
        }
      }
      frame "CAMERA_define_ROI" {
        n79 = Variant To Data(error in=w293, type=T7 {"Sub Region"={"Horizontal Offset"=0, "Vertical Offset"=0, "Horizontal Size"=0, "Vertical Size"=0}, "Start acquisition"=FALSE} ("output cluster"), Variant=w294) -> (data=w291:T7, error out=w292:errorcluster)
        n80 = Unbundle By Name(w291) -> ("Sub Region"=w276:T14, "Start acquisition"=w288:bool)
        n81 = call "CAMERA_task_START.vi"("error in"=w292) -> ("error out"=w290:errorcluster)
        n82 = case shown="True" w288 {
          tunnel: [w305 w307] -> w280
          tunnel: w290 -> [w305 w311]
          tunnel: w285 -> [w304 w310]
          tunnel: [w304 w306] -> w278
          frame False {
          }
          frame True {
            n83 = call <userlib>:"tm_stopcapture_40.vi"("error in (no error)"=w311, "Handle in"=w310) -> ("error out"=w309:errorcluster, "Handle out"=w308:u32)  [unwired: 8 in]
            n84 = call <userlib>:"tm_unpreparecapture_40.vi"("error in (no error)"=w309, "Handle in"=w308) -> ("error out"=w307:errorcluster, "Handle out"=w306:u32)  [unwired: 8 in]
          }
        }
        n85 = call <userlib>:"tm_setarea_40.vi"("error in (no error)"=w280, "Sub Region"=w276, "Handle in"=w278) -> ("error out"=w279:errorcluster, "Handle out"=w277:u32)  [unwired: 7 in]
        n86 = case shown="True" w288 {
          tunnel: w279 -> [w295 w301]
          tunnel: [w295 w296] -> w282
          tunnel: w277 -> [_ w300]
          frame False {
          }
          frame True {
            w299 = 1 items=["Snap", "Sequence"] ("Capture mode")
            n87 = call <userlib>:"tm_preparecapture_40.vi"("error in (no error)"=w301, "Capture mode"=w299, "Handle in"=w300) -> ("error out"=w298:errorcluster, "Handle out"=w297:u32)  [unwired: 5 in, 2 out]
            n88 = call <userlib>:"tm_startcapture_40.vi"("error in (no error)"=w298, "Handle in"=w297) -> ("error out"=w296:errorcluster)  [unwired: 8 in, 1 out]
          }
        }
        n89 = call "CAMERA_task_DONE.vi"("error in"=w282) -> ("error out"=w289:errorcluster)
        n90 = case shown="False" w288 {
          tunnel: [T3 {"variant"=variant, "Instruction"=enum."CAMERA_not_acquiring"} ("Q_ANDOR_element") T3 {"variant"=variant, "Instruction"=enum."CAMERA_acquiring"} ("Q_ANDOR_element")] -> w287
          frame False {
          }
          frame True {
          }
        }
      }
      frame "CAMERA_cooler" {
        w316 = u32 2115280 items=["SENSOR MODE"=4212128, "READOUT SPEED"=4211872, "READOUT DIRECTION"=4211904, "TRIGGER GLOBAL EXPOSURE"=2049680, "TRIGGER DELAY"=1066480, "INTERNAL TRIGGER HANDLING"=1066496, "SYNC READOUT SYSTEM BLANK"=1066528, "SENSOR TEMPERATURE"=2115232, "SENSOR COOLER STATUS"=2115280, "EXPOSURE TIME"=2049184, "DEFECT CORRECT MODE"=4670368, "BINNING"=4215968, "INTERNAL LINE SPEED"=4226000, "INTERNAL LINE INTERVAL"=4226016, "NUMBER OF OUTPUT TRIGGER CONNECTOR"=1852320, "OUTPUT TRIGGER SOURCE[0]"=1852576, "OUTPUT TRIGGER SOURCE[1]"=1852832, "OUTPUT TRIGGER SOURCE[2]"=1853088, "OUTPUT TRIGGER POLARITY[0]"=1852592, "OUTPUT TRIGGER POLARITY[1]"=1852848, "OUTPUT TRIGGER POLARITY[2]"=1853104, "OUTPUT TRIGGER ACTIVE[0]"=1852608, "OUTPUT TRIGGER ACTIVE[1]"=1852864, "OUTPUT TRIGGER ACTIVE[2]"=1853120, "OUTPUT TRIGGER DELAY[0]"=1852624, "OUTPUT TRIGGER DELAY[1]"=1852880, "OUTPUT TRIGGER DELAY[2]"=1853136, "OUTPUT TRIGGER PERIOD[0]"=1852640, "OUTPUT TRIGGER PERIOD[1]"=1852896, "OUTPUT TRIGGER PERIOD[2]"=1853152, "OUTPUT TRIGGER KIND[0]"=1852656, "OUTPUT TRIGGER KIND[1]"=1852912, "OUTPUT TRIGGER KIND[2]"=1853168, "OUTPUT TRIGGER BASE SENSOR[0]"=1852672, "OUTPUT TRIGGER BASE SENSOR[1]"=1852928, "OUTPUT TRIGGER BASE SENSOR[2]"=1853184, "OUTPUT TRIGGER PRE HSYNC COUNT"=1852704] ("Parameter")
        n91 = call "CAMERA_task_START.vi"("error in"=w328) -> ("error out"=w324:errorcluster)
        n92 = Variant To Data(error in=w324, type=FALSE ("Cooler"), Variant=w327) -> (data=w321:bool, error out=w318:errorcluster)
        n93 = Select(t=1.0, s=w321, f=2.0) -> (s? t:f=w317:dbl)
        n94 = call <userlib>:"tm_setparameter_40.vi"("error in (no error)"=w318, "Value in"=w317, "Parameter"=w316, "Handle in"=w314) -> ("error out"=w313:errorcluster)  [unwired: 6 in, 1 out]
        n95 = call "CAMERA_task_DONE.vi"("error in"=w313) -> ("error out"=w323:errorcluster)
      }
      frame "CAMERA_acquire_movie" {
        n96 = call "CAMERA_task_START.vi"("error in"=w347) -> ("error out"=w331:errorcluster)
        n97 = Variant To Data(error in=w331, type=T9 {"Saving path"=path "", "Sample name"="", "N frames"=0, "N movies"=0, "Start acquisition"=FALSE, "Global parameters"={"405"=0.0, "488"=0.0, "561"=0.0, "641"=0.0, "BF"=0.0, "X"=0.0, "Y"=0.0, "Filter list"=0, "Exp time"=0.0, "Kinetic time"=0.0, "Gain"=0, "Step length (nm)"=0, "Total range (nm)"=0, "Scan illumination\n mode"=FALSE, "Dt (s)"=0, "# repetitions"=0}} ("output cluster"), Variant=w352) -> (data=w337:T9, error out=w335:errorcluster)
        n98 = Unbundle By Name(w337) -> ("Global parameters"=w338:T8, "N movies"=w343:i32, "N frames"=w341:i32)
        n99 = Unbundle By Name(w337) -> ("Start acquisition"=w330:bool, "Saving path"=w334:path, "Sample name"=w332:string)
        n100 = call "MOVIE_save_path_folder_definition.vi"("error in"=w335, "Sample name"=w332, "Path to the saving folder"=w334) -> ("error out"=w336:errorcluster, "Movie folder"=w329:string, "Parameter path"=w333:path)  [unwired: 3 in]
        n101 = for {
          N: w343 -> [_]
          tunnel: w349 -> [w370]
          tunnel: w336 -> [w367]
          tunnel: [w359] -> w348
          tunnel: w339 -> [w366]
          tunnel: w341 -> [w354]
          tunnel: w339 -> [w363]
          tunnel: w329 -> [w356]
          tunnel: w330 -> [w355]
          i -> [w353]
          n102 = call "MOVIE_setup_acquisition_sCMOS.vi"("frames"=w354, "Handle in"=w366, "Acquiring"=w355, "Movie folder name"=w356, "Movie number"=w353, "error in"=w367) -> ("t0"=w357:dbl, "error out"=w358:errorcluster)  [unwired: 1 in]
          n103 = global write "Global_CAMERA.vi" "Frames acquired"(w353) -> ()
          n104 = while {
            tunnel: w358 -> [w383]
            tunnel: [w382] -> w362
            tunnel: w370 -> [w381]
            shift-right: [w377] -> _
            shift-left: -1 ("Frames acquired out") -> [w380]
            shift-right: [w378] -> _
            shift-left: 0 ("N repeat out") -> [w379]
            tunnel: w354 -> [w373]
            tunnel: w357 -> [w372]
            stop <- w375 stop-if-true
            n105 = call "sCMOS_acquire_Save_movie.vi"("t0"=w372, "Frames acquired"=w380, "N repeat"=w379, "error in"=w383, "Image IN"=w381, "Number of images"=w373) -> ("Stop?"=w376:bool, "Frames acquired out"=w377:i32, "N repeat out"=w378:i32, "error out"=w382:errorcluster)  [unwired: 10 in]
            n106 = global read "Global_ABORT.vi" "ABORT"() -> (w374:bool)
            n107 = Wait (ms)(milliseconds to wait=u32 1) -> ()  [unwired: 1 out]
            n108 = Or(x=w376, y=w374) -> (x .or. y?=w375:bool)
          }
          n109 = call <userlib>:"tm_stoprecorder_40.vi"("error in (no error)"=w362, "Handle in"=w363) -> ("error out"=w365:errorcluster, "Handle out"=w364:u32)  [unwired: 8 in]
          n110 = call <userlib>:"tm_stopcapture_40.vi"("error in (no error)"=w365, "Handle in"=w364) -> ("error out"=w360:errorcluster, "Handle out"=w361:u32)  [unwired: 8 in]
          n111 = call <userlib>:"tm_unpreparecapture_40.vi"("error in (no error)"=w360, "Handle in"=w361) -> ("error out"=w359:errorcluster)  [unwired: 8 in, 1 out]
        }
        n112 = call "MOVIE_close_movie_acquisition_sCMOS.vi"("error in"=w348, "parameters path"=w333, "Global parameters"=w338) -> ("error out"=w346:errorcluster)  [unwired: 1 in]
        n113 = call "CAMERA_task_DONE.vi"("error in"=w346) -> ("error out"=w345:errorcluster)
      }
      frame "CAMERA_init_scan" {
        n114 = call "CAMERA_task_START.vi"("error in"=w398) -> ("error out"=w393:errorcluster)
        n115 = Flush Queue(queue=w391, error in (no error)=w393) -> (error out=w392:errorcluster)  [unwired: 2 out]
        n116 = Variant To Data(error in=w392, type=T10 {"Frames"=0, "Movie path"=path "", "Start acquisition"=FALSE} ("output cluster"), Variant=w399) -> (data=w387:T10, error out=w389:errorcluster)
        n117 = call "sCMOS_init_ramp.vi"("error in"=w389, "data cluster"=w387, "handle"=w386) -> ("error out"=w384:errorcluster, "Ready?"=w385:bool)  [unwired: 1 in]
        n118 = global write "Global_CAMERA.vi" "CAMERA ready"(w385) -> ()
        n119 = call "CAMERA_task_DONE.vi"("error in"=w384) -> ("error out"=w397:errorcluster)
      }
      frame "CAMERA_check_new_scan_image" {
        # "During the scan, at each step an internal software trigger is sent by the camera to the camera. This step is used to initiate the acquisition of a single image. Since the acquisition is not instantaneous, the program is waiting in a while loop and at each iteration it:\n\n- checks whether the new image is acquired\n- the abort control was not activated\n- the time spent in the loop is not too long (three times the expected acquisition time). \n\nIf one of the three possibilities is checked, the while loop is stopped and the program proceeds."
        n120 = call "CAMERA_task_START.vi"("error in"=w424) -> ("error out"=w404:errorcluster)
        n121 = call <userlib>:"tm_firetrigger_40.vi"("error in (no error)"=w404, "Handle in"=w400) -> ("error out"=w405:errorcluster)  [unwired: 8 in, 1 out]
        n122 = Variant To Data(error in=w405, type=T11 {"Pulse length Ton (s)"=0.0, "image #"=0, "Display?"=FALSE} ("output cluster"), Variant=w423) -> (data=w402:T11, error out=w422:errorcluster)
        n123 = Unbundle By Name(w402) -> ("Display?"=w401:bool)
        n124 = Unbundle By Name(w402) -> ("image #"=w412:i32, "Pulse length Ton (s)"=w409:dbl)
        n125 = flat-sequence {
          tunnel: w422 -> [w455]
          tunnel: [w455] -> w414
          tunnel: [w454] -> w413
          frame #0 {
            n126 = call <vilib>:"High Resolution Relative Seconds.vi"() -> ("relative seconds"=w454:dbl)
          }
        }
        n127 = Multiply(x=w409, y=3.0) -> (x*y=w408:dbl)
        n128 = while {
          tunnel: w414 -> [w443]
          tunnel: w413 -> [w452]
          tunnel: w412 -> [w439]
          tunnel: [w446] -> w411
          tunnel: [w442] -> w410
          tunnel: w408 -> [w444]
          tunnel: w400 -> [w440]
          tunnel: [w438] -> w406
          stop <- w447 stop-if-true
          n129 = call <vilib>:"High Resolution Relative Seconds.vi"() -> ("relative seconds"=w453:dbl)
          n130 = call <userlib>:"tm_getcaptureinfo_40.vi"("error in (no error)"=w443, "Handle in"=w440) -> ("error out"=w442:errorcluster, "Frame Count"=w441:i32, "Frame Index"=w438:i32)  [unwired: 6 in, 1 out]
          n131 = global read "Global_ABORT.vi" "ABORT"() -> (w450:bool)
          n132 = Subtract(x=w453, y=w452) -> (x-y=w451:dbl)
          n133 = Equal?(x=w439, y=w441) -> (x = y?=w446:bool)
          n134 = Less?(x=w444, y=w451) -> (x < y?=w449:bool)
          n135 = Wait (ms)(milliseconds to wait=u32 5) -> ()  [unwired: 1 out]
          n136 = Build Array(w450, w446, w449) -> (w448:bool[])
          n137 = Or Array Elements(Boolean array=w448) -> (logical OR=w447:bool)
        }
        n138 = case shown="True" w411 {
          tunnel: w410 -> [w426 w435]
          tunnel: w421 -> [_ w432]
          tunnel: [w425 w433] -> w420
          tunnel: w400 -> [_ w431]
          tunnel: w406 -> [_ w430]
          tunnel: w401 -> [_ w429]
          frame False {
            n139 = flat-sequence {
              tunnel: w426 -> [w428]
              tunnel: [w428] -> w425
              frame #0 {
                n140 = global write "Global_CAMERA.vi" "CAMERA ready"(FALSE ("ANDOR ready")) -> ()
              }
            }
          }
          frame True {
            n141 = call "sCMOS_get_last_image.vi"("Display?"=w429, "Image In"=w432, "Frame Index"=w430, "Error in"=w435, "Handle in"=w431) -> ("image error"=w434:errorcluster)  [unwired: 1 in]
            n142 = flat-sequence {
              tunnel: w434 -> [w437]
              tunnel: [w437] -> w433
              frame #0 {
                n143 = global write "Global_CAMERA.vi" "CAMERA ready"(TRUE ("ANDOR ready")) -> ()
              }
            }
          }
        }
        n144 = call "CAMERA_task_DONE.vi"("error in"=w420) -> ("error out"=w416:errorcluster)
      }
      frame "CAMERA_close_scan" {
        n145 = call "CAMERA_task_START.vi"("error in"=w474) -> ("error out"=w457:errorcluster)
        n146 = call <userlib>:"tm_stoprecorder_40.vi"("error in (no error)"=w457, "Handle in"=w456) -> ("error out"=w459:errorcluster, "Handle out"=w458:u32)  [unwired: 8 in]
        n147 = call <userlib>:"tm_stopcapture_40.vi"("error in (no error)"=w459, "Handle in"=w458) -> ("error out"=w468:errorcluster, "Handle out"=w469:u32)  [unwired: 8 in]
        n148 = call <userlib>:"tm_unpreparecapture_40.vi"("error in (no error)"=w468, "Handle in"=w469) -> ("error out"=w466:errorcluster, "Handle out"=w467:u32)  [unwired: 8 in]
        n149 = call <userlib>:"tm_setinputtrigger_40.vi"("error in (no error)"=w466, "Parameters"=T12 {"Mode"=1, "Polarity"=1, "Times"=1, "Delay"=0.0}, "Handle in"=w467) -> ("error out"=w463:errorcluster, "Handle out"=w464:u32)  [unwired: 7 in]
        n150 = call <userlib>:"tm_setoutputtrigger_40.vi"("Port"=1, "error in (no error)"=w463, "Type"=cluster{"Mode":u32, "Polarity":u32} {"Mode"=1, "Polarity"=1}, "Handle in"=w464) -> ("error out"=w461:errorcluster)  [unwired: 6 in, 1 out]
        n151 = call "CAMERA_task_DONE.vi"("error in"=w461) -> ("error out"=w475:errorcluster)
      }
      frame "CAMERA_init_merFISH" {
        n152 = call "CAMERA_task_START.vi"("error in"=w490) -> ("error out"=w485:errorcluster)
        n153 = Flush Queue(queue=w483, error in (no error)=w485) -> (error out=w484:errorcluster)  [unwired: 2 out]
        n154 = Variant To Data(error in=w484, type=FALSE, Variant=w491) -> (data=w476:bool, error out=w480:errorcluster)
        n155 = call "sCMOS_init_merFISH.vi"("error in"=w480, "Start acquisition"=w476, "handle"=w479) -> ("error out"=w478:errorcluster)  [unwired: 2 in]
        n156 = case shown="No Error" w478 {
          selector: w478 -> [w493 w495]
          tunnel: [w493 w495] -> w488
          frame Error {
            n157 = global write "Global_CAMERA.vi" "CAMERA ready"(FALSE ("ANDOR ready")) -> ()
          }
          frame No Error {
            n158 = global write "Global_CAMERA.vi" "CAMERA ready"(TRUE ("ANDOR ready")) -> ()
          }
        }
        n159 = call "CAMERA_task_DONE.vi"("error in"=w488) -> ("error out"=w489:errorcluster)
      }
      frame "CAMERA_start_acquiring_merFISH" {
        n160 = call "CAMERA_task_START.vi"("error in"=w510) -> ("error out"=w509:errorcluster)
        n161 = Flush Queue(queue=w512, error in (no error)=w509) -> (error out=w508:errorcluster)  [unwired: 2 out]
        n162 = Variant To Data(error in=w508, type=cluster{"Movie path":path, "Total # frames":i32} {"Movie path"=path "", "Total # frames"=0} ("output cluster"), Variant=w507) -> (data=w504:cluster{"Movie path":path, "Total # frames":i32}, error out=w506:errorcluster)
        n163 = Unbundle By Name(w504) -> ("Movie path"=w502:path, "Total # frames"=w503:i32)
        n164 = call <userlib>:"tm_startrecorder_40.vi"("error in (no error)"=w506, "frames"=w503, "File"=w502, "Handle in"=w496) -> ("error out"=w498:errorcluster, "Handle out"=w500:u32)  [unwired: 6 in]
        n165 = flat-sequence {
          tunnel: w500 -> [w519]
          tunnel: [w519] -> w499
          tunnel: w498 -> [w518]
          tunnel: [w518] -> w497
          frame #0 {
            n166 = Wait (ms)(milliseconds to wait=u32 1000) -> ()  [unwired: 1 out]
          }
        }
        n167 = call <userlib>:"tm_startcapture_40.vi"("error in (no error)"=w497, "Handle in"=w499) -> ("error out"=w501:errorcluster)  [unwired: 8 in, 1 out]
        n168 = call "CAMERA_task_DONE.vi"("error in"=w501) -> ("error out"=w513:errorcluster)
      }
      frame "CAMERA_close_scan_merFISH" {
        n169 = call "CAMERA_task_START.vi"("error in"=w529) -> ("error out"=w523:errorcluster)
        n170 = call <userlib>:"tm_stoprecorder_40.vi"("error in (no error)"=w523, "Handle in"=w520) -> ("error out"=w522:errorcluster, "Handle out"=w521:u32)  [unwired: 8 in]
        n171 = call <userlib>:"tm_stopcapture_40.vi"("error in (no error)"=w522, "Handle in"=w521) -> ("error out"=w524:errorcluster)  [unwired: 8 in, 1 out]
        n172 = call "CAMERA_task_DONE.vi"("error in"=w524) -> ("error out"=w530:errorcluster)
      }
      frame "CAMERA_close_merFISH" {
        n173 = call "CAMERA_task_START.vi"("error in"=w548) -> ("error out"=w534:errorcluster)
        n174 = call <userlib>:"tm_stopcapture_40.vi"("error in (no error)"=w534, "Handle in"=w532) -> ("error out"=w542:errorcluster, "Handle out"=w543:u32)  [unwired: 8 in]
        n175 = call <userlib>:"tm_unpreparecapture_40.vi"("error in (no error)"=w542, "Handle in"=w543) -> ("error out"=w540:errorcluster, "Handle out"=w541:u32)  [unwired: 8 in]
        n176 = call <userlib>:"tm_setinputtrigger_40.vi"("error in (no error)"=w540, "Parameters"=T12 {"Mode"=1, "Polarity"=1, "Times"=1, "Delay"=0.0}, "Handle in"=w541) -> ("error out"=w537:errorcluster, "Handle out"=w538:u32)  [unwired: 7 in]
        n177 = call <userlib>:"tm_setoutputtrigger_40.vi"("Port"=1, "error in (no error)"=w537, "Type"=cluster{"Mode":u32, "Polarity":u32} {"Mode"=1, "Polarity"=1}, "Handle in"=w538) -> ("error out"=w533:errorcluster)  [unwired: 6 in, 1 out]
        n178 = flat-sequence {
          tunnel: w533 -> [w551]
          tunnel: [w551] -> w545
          frame #0 {
            n179 = global write "Global_CAMERA.vi" "CAMERA ready"(FALSE ("ANDOR ready")) -> ()
          }
        }
        n180 = call "CAMERA_task_DONE.vi"("error in"=w545) -> ("error out"=w549:errorcluster)
      }
      frame "CAMERA_init_TL" {
        n181 = call "CAMERA_task_START.vi"("error in"=w566) -> ("error out"=w561:errorcluster)
        n182 = Flush Queue(queue=w559, error in (no error)=w561) -> (error out=w560:errorcluster)  [unwired: 2 out]
        n183 = Variant To Data(error in=w560, type=TRUE, Variant=w567) -> (data=w552:bool, error out=w556:errorcluster)
        n184 = call "sCMOS_init_TL.vi"("error in"=w556, "Start acquisition"=w552, "handle"=w555) -> ("error out"=w554:errorcluster)  [unwired: 2 in]
        n185 = case shown="No Error" w554 {
          selector: w554 -> [w569 w571]
          tunnel: [w569 w571] -> w564
          frame Error {
            n186 = global write "Global_CAMERA.vi" "CAMERA ready"(FALSE ("ANDOR ready")) -> ()
          }
          frame No Error {
            n187 = global write "Global_CAMERA.vi" "CAMERA ready"(TRUE ("ANDOR ready")) -> ()
          }
        }
        n188 = call "CAMERA_task_DONE.vi"("error in"=w564) -> ("error out"=w565:errorcluster)
      }
      frame "CAMERA_start_acquiring_TL" {
        n189 = call "CAMERA_task_START.vi"("error in"=w591) -> ("error out"=w583:errorcluster)
        n190 = Variant To Data(error in=w583, type=cluster{"N Frames":i32, "movie path":path} {"N Frames"=0, "movie path"=path ""} ("output cluster"), Variant=w582) -> (data=w580:cluster{"N Frames":i32, "movie path":path}, error out=w577:errorcluster)
        n191 = Unbundle By Name(w580) -> ("movie path"=w579:path, "N Frames"=w578:i32)
        n192 = call <userlib>:"tm_startrecorder_40.vi"("error in (no error)"=w577, "frames"=w578, "File"=w579, "Handle in"=w576) -> ("error out"=w573:errorcluster, "Handle out"=w575:u32)  [unwired: 6 in]
        n193 = flat-sequence {
          tunnel: w575 -> [w594]
          tunnel: [w594] -> w574
          tunnel: w573 -> [w593]
          tunnel: [w593] -> w572
          frame #0 {
            n194 = Wait (ms)(milliseconds to wait=u32 1000) -> ()  [unwired: 1 out]
          }
        }
        n195 = call <userlib>:"tm_startcapture_40.vi"("error in (no error)"=w572, "Handle in"=w574) -> ("error out"=w584:errorcluster)  [unwired: 8 in, 1 out]
        n196 = case shown="Error" w584 {
          selector: w584 -> [w596 w598]
          tunnel: [w596 w598] -> w589
          frame Error {
            n197 = global write "Global_CAMERA.vi" "CAMERA ready"(FALSE ("ANDOR ready")) -> ()
          }
          frame No Error {
            n198 = global write "Global_CAMERA.vi" "CAMERA ready"(TRUE ("ANDOR ready")) -> ()
          }
        }
        n199 = call "CAMERA_task_DONE.vi"("error in"=w589) -> ("error out"=w590:errorcluster)
      }
      frame "CAMERA_stop_acquiring_TL" {
        n200 = call "CAMERA_task_START.vi"("error in"=w610) -> ("error out"=w602:errorcluster)
        n201 = call <userlib>:"tm_stoprecorder_40.vi"("error in (no error)"=w602, "Handle in"=w603) -> ("error out"=w601:errorcluster, "Handle out"=w600:u32)  [unwired: 8 in]
        n202 = call <userlib>:"tm_stopcapture_40.vi"("error in (no error)"=w601, "Handle in"=w600) -> ("error out"=w599:errorcluster)  [unwired: 8 in, 1 out]
        n203 = case shown="Error" w599 {
          selector: w599 -> [w612 w614]
          tunnel: [w612 w614] -> w608
          frame Error {
            n204 = global write "Global_CAMERA.vi" "CAMERA ready"(FALSE ("ANDOR ready")) -> ()
          }
          frame No Error {
            n205 = global write "Global_CAMERA.vi" "CAMERA ready"(FALSE ("ANDOR ready")) -> ()
          }
        }
        n206 = call "CAMERA_task_DONE.vi"("error in"=w608) -> ("error out"=w609:errorcluster)
      }
      frame "CAMERA_close_TL" {
        n207 = call "CAMERA_task_START.vi"("error in"=w632) -> ("error out"=w618:errorcluster)
        n208 = call <userlib>:"tm_stopcapture_40.vi"("error in (no error)"=w618, "Handle in"=w616) -> ("error out"=w626:errorcluster, "Handle out"=w627:u32)  [unwired: 8 in]
        n209 = call <userlib>:"tm_unpreparecapture_40.vi"("error in (no error)"=w626, "Handle in"=w627) -> ("error out"=w624:errorcluster, "Handle out"=w625:u32)  [unwired: 8 in]
        n210 = call <userlib>:"tm_setinputtrigger_40.vi"("error in (no error)"=w624, "Parameters"=T12 {"Mode"=1, "Polarity"=1, "Times"=1, "Delay"=0.0}, "Handle in"=w625) -> ("error out"=w621:errorcluster, "Handle out"=w622:u32)  [unwired: 7 in]
        n211 = call <userlib>:"tm_setoutputtrigger_40.vi"("Port"=1, "error in (no error)"=w621, "Type"=cluster{"Mode":u32, "Polarity":u32} {"Mode"=1, "Polarity"=1}, "Handle in"=w622) -> ("error out"=w617:errorcluster)  [unwired: 6 in, 1 out]
        n212 = flat-sequence {
          tunnel: w617 -> [w635]
          tunnel: [w635] -> w629
          frame #0 {
            n213 = global write "Global_CAMERA.vi" "CAMERA ready"(FALSE ("ANDOR ready")) -> ()
          }
        }
        n214 = call "CAMERA_task_DONE.vi"("error in"=w629) -> ("error out"=w633:errorcluster)
      }
      frame "CAMERA_STOP" {
        n215 = call "CAMERA_task_START.vi"("error in"=w650) -> ("error out"=w643:errorcluster)
        n216 = Flush Queue(queue=w636, error in (no error)=w643) -> (error out=w637:errorcluster)  [unwired: 2 out]
        n217 = call "IMAQ Dispose"("Image"=w647, "error in (no error)"=w637) -> ("error out"=w641:errorcluster)  [unwired: 4 in]
        n218 = Variant To Data(error in=w641, type=FALSE, Variant=w640) -> (data=w638:bool, error out=w639:errorcluster)
        n219 = case shown="True" w638 {
          tunnel: w645 -> [w657 w664]
          tunnel: [w659 w662] -> w644
          tunnel: w639 -> [w658 w661]
          frame True {
            n220 = call <userlib>:"tm_stopcapture_40.vi"("error in (no error)"=w658, "Handle in"=w657) -> ("error out"=w656:errorcluster, "Handle out"=w654:u32)  [unwired: 8 in]
            n221 = call <userlib>:"tm_unpreparecapture_40.vi"("error in (no error)"=w656, "Handle in"=w654) -> ("error out"=w655:errorcluster, "Handle out"=w653:u32)  [unwired: 8 in]
            n222 = call <userlib>:"tm_closecamera_40.vi"("error in (no error)"=w655, "Handle in"=w653) -> ("error out"=w660:errorcluster)  [unwired: 9 in]
            n223 = call <userlib>:"tm_deinitialize_40.vi"("error in (no error)"=w660) -> ("error out"=w659:errorcluster)  [unwired: 10 in]
          }
          frame False {
            n224 = call <userlib>:"tm_closecamera_40.vi"("error in (no error)"=w661, "Handle in"=w664) -> ("error out"=w663:errorcluster)  [unwired: 9 in]
            n225 = call <userlib>:"tm_deinitialize_40.vi"("error in (no error)"=w663) -> ("error out"=w662:errorcluster)  [unwired: 10 in]
          }
        }
        n226 = call "CAMERA_task_DONE.vi"("error in"=w644) -> ("error out"=w648:errorcluster)
      }
    }
    n227 = global read "Global_MAIN.vi" "Stop main vi"() -> (w51:bool)
    n228 = To Variant(anything=w33) -> (Variant=w34:variant)
    n229 = Bundle By Name(cluster=T3 {"variant"=variant, "Instruction"=enum."CAMERA_error"} ("Q_ANDOR_element"), "variant"=w34) -> (w32:T3)
    n230 = case shown="No Error" w33 {
      selector: w33 -> [w52 _]
      tunnel: w45 -> [w56 _]
      tunnel: [w55 w60] -> w44
      tunnel: [w54 w59] -> w36
      tunnel: w25 -> [w53 w58]
      tunnel: w32 -> [_ w57]
      frame No Error {
        n231 = Enqueue Element(queue=w53, element=w56, error in (no error)=w52) -> (queue out=w55:refnum<queue>, error out=w54:errorcluster)  [unwired: 1 in, 1 out]
      }
      frame Error {
        n232 = Enqueue Element(queue=w58, element=w57) -> (queue out=w60:refnum<queue>, error out=w59:errorcluster)  [unwired: 2 in, 1 out]
      }
    }
    n233 = Wait (ms)(milliseconds to wait=u32 10) -> ()  [unwired: 1 out]
  }
  n234 = flat-sequence {
    tunnel: FALSE ("Stop main vi") -> [w665]
    tunnel: [w665] -> w7
    frame #0 {
      n235 = global write "Global_CAMERA.vi" "Frames acquired"(0 ("Frames acquired")) -> ()
      n236 = global write "Global_ABORT.vi" "ABORT"(w665) -> ()
      n237 = global write "Global_MAIN.vi" "Stop main vi"(w665) -> ()
      n238 = global write "Global_CAMERA.vi" "CAMERA done"(w665) -> ()
      n239 = global write "Global_CAMERA.vi" "Start CAMERA"(w665) -> ()
      n240 = global write "Global_CAMERA.vi" "CAMERA ready"(w665) -> ()
    }
  }
  n241 = Release Queue(queue=w6, error in (no error)=w5) -> ()  [unwired: 1 in, 3 out]
